vi "To Path Tree Data.vi"(10 "Path":path) -> (3 "Path Tree Data":refnum<class "Path.lvclass">)   [LabVIEW 2017, in "Tree API.lvlib" / "Path.lvclass"]
doc: "Convert a Path value to Tree Data type."
uses:
  Path.lvclass
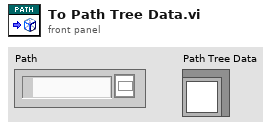
[diagram p1: front panel]
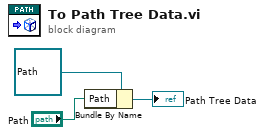
[diagram p0: block diagram]
diagram:
  n1 = Bundle By Name(cluster=refnum<class "Path.lvclass"> refnum ("Path in"), "Path"="Path") -> (→"Path Tree Data":refnum<class "Path.lvclass">)
